vi "WILT Array Insert on Bottom.vi"(7 "Max Num Records":i32=50, 10 "New String":string, 11 "appended array":string[][](array[string])) -> (3 "output array":string[][](array[string]))   [LabVIEW 2016]
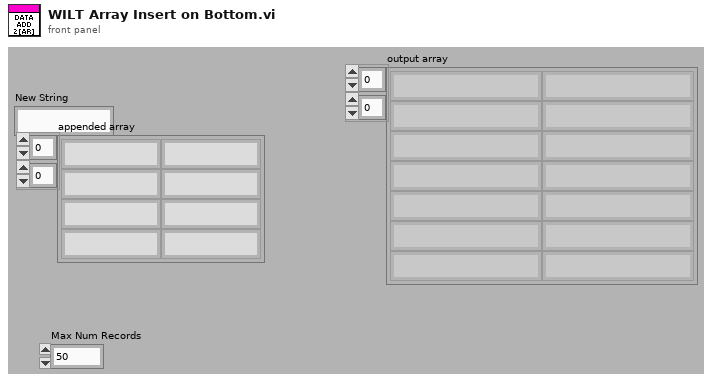
[diagram p1: front panel]
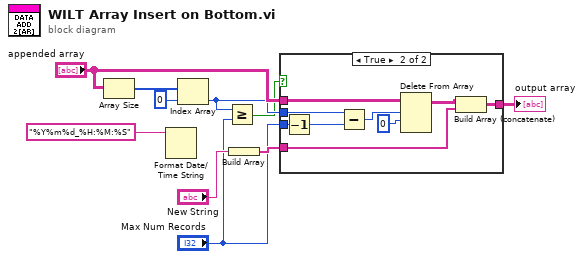
[diagram p0: block diagram]
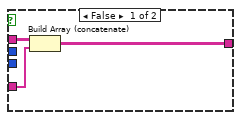
[diagram p2: hidden frame]
diagram:
  n1 = Array Size(array="appended array") -> (size(s)=w9:i32[])
  n2 = Format Date/Time String(time format string (%c)="%Y%m%d_%H:%M:%S") -> ()  [unwired: 3 out]
  n3 = Index Array(array=w9, index=0) -> (element=w6:i32)
  n4 = Greater Or Equal?(x=w6, y="Max Num Records") -> (x >= y?=w3:bool)
  n5 = Build Array("New String") -> (w5:string[])
  n6 = case shown="True" w3 {
    tunnel: "appended array" -> [w13 w22]
    tunnel: w6 -> [_ w20]
    tunnel: w5 -> [w12 w15]
    tunnel: [w11 w17] -> w4
    tunnel: "Max Num Records" -> [_ w18]
    frame False {
      n7 = Build Array (concatenate)(w13, w12) -> (w11:string[][])
    }
    frame True {
      n8 = Decrement(x=w18) -> (x-1=w14:i32)
      n9 = Subtract(x=w20, y=w14) -> (x-y=w21:i32)
      n10 = Delete From Array(array=w22, length=w21, index (row)=0) -> (array with subset deleted=w16:string[][])  [unwired: 1 in, 1 out]
      n11 = Build Array (concatenate)(w16, w15) -> (w17:string[][])
    }
  }
  "output array" <- w4
